vi "Configure Number of Averages.vi"(8 "error in (no error)":errorcluster {"code" format="%.0x"}, 10 "Number of Averages (8)":i32=8, 11 "VISA Resource Name":refnum<visa-resource-name>) -> (0 "error out":errorcluster {"code" format="%.0x"}, 3 "VISA Resource Name Out":refnum<visa-resource-name>)   [LabVIEW 2011, in "Agilent 546XX Series.lvlib"]
doc: "This VI configures the number of waveforms that the oscilloscope acquires and averages. After the oscilloscope acquires as many waveforms as you specify, it returns to the idle state. \n\nNotes:\n\n(1) Set the acquisition type to Average before you call this VI. To set the acquisition type, call the ag546xx Configure Acquisition Type VI."
uses:
  Agilent 546XX Series.lvlib
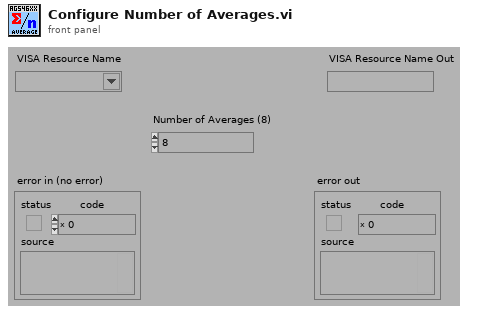
[diagram p1: front panel]
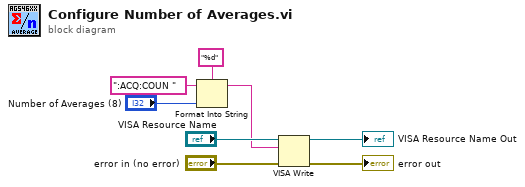
[diagram p0: block diagram]
diagram:
  n1 = Format Into String(format string="%d", initial string=":ACQ:COUN ", "Number of Averages (8)") -> (resulting string=w1:string)  [unwired: 1 in, 1 out]
  n2 = VISA Write(VISA resource name="VISA Resource Name", write buffer=w1, error in (no error)="error in (no error)") -> (VISA resource name out=→"VISA Resource Name Out":refnum<visa-resource-name>, error out=→"error out":errorcluster)  [unwired: 1 out]
